vi "applyInsertSpace.vi"(4 "deltaY":u16, 6 "deltaX":u16, 8 "error in (no error)":errorcluster, 10 "origin":T1, 11 "Wire in":refnum<class "Wire.lvclass">) -> (0 "error out":errorcluster, 3 "Wire out":refnum<class "Wire.lvclass">)   [LabVIEW 2023, in "TLC_Scripto.lvlib" / "Wire.lvclass"]
uses:
  Wire.lvclass
  Wire.lvclass/Wire.ctl
  Ctrls/point.ctl
  TLC_Scripto.lvlib
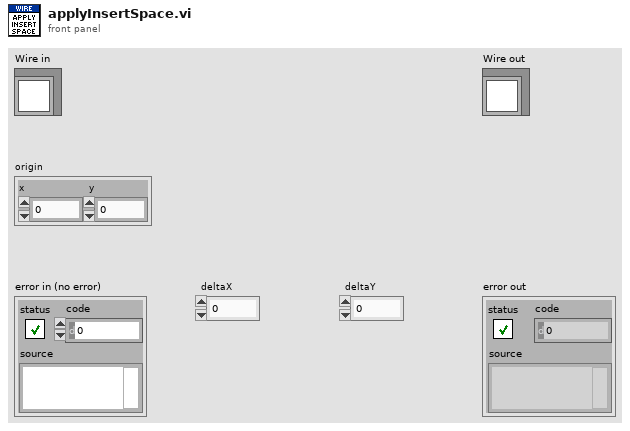
[diagram p1: front panel]
types:
  T1 = typedef "TLC_Scripto.lvlib/point.ctl" = cluster{"x":i32, "y":i32}
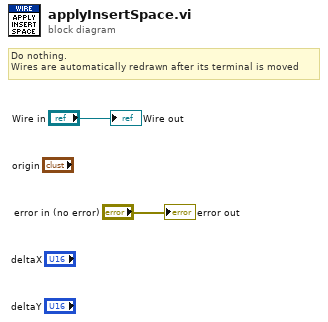
[diagram p0: block diagram]
diagram:
  # "Do nothing.\nWires are automatically redrawn after its terminal is moved"
  "error out" <- "error in (no error)"
  "Wire out" <- "Wire in"
